vi "util.file.vars.vi"(4 "Operation(Read)":enum16{"Read File", "Write File"}(ring), 6 "allowDialogs?(False)":bool, 8 "error in":errorcluster, 9 "Directory (DIR_PROC)":T1, 10 "Proc Name(open dialog if empty)":string, 11 "Vars[] in":variant[](array[variant])) -> (0 "error out":errorcluster, 1 "filename":string, 2 "cancelled?":bool, 3 "Vars[] out":variant[](array[variant]), 5 "File path":path)   [LabVIEW 2024]
uses:
  controls/typePathSelector.ctl
  controls/typeProcVarientName.ctl
  Polymorphics/variantCtrlString.vi
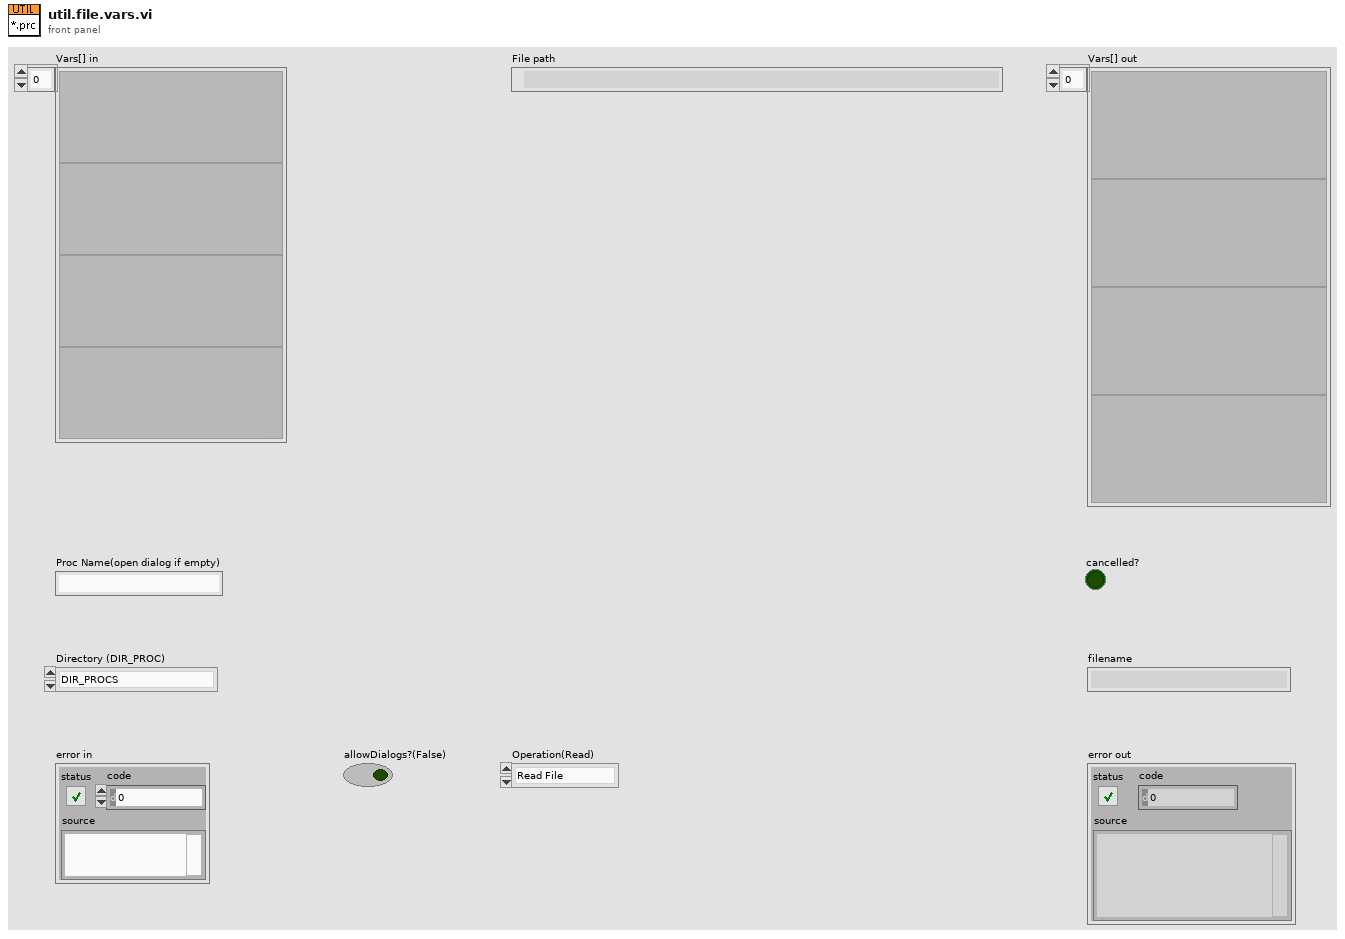
[diagram p1: front panel]
types:
  T1 = typedef "typePathSelector.ctl" = enum16{"DIR_PROCS", "DIR_CONFIG", "DIR_TEMPLATE", "DIR_IO_FILE", "DIR_RECORD", "DIR_LOG", "DIR_RUNTIME", "DIR_PRESET", "DIR_INI"}
  T2 = typedef "typeProcVarientName.ctl" = enum16{"procNameID", "procModuleID", "procPath", "procIsRunning", "procIndex", "procModule", "procRegisterNumeric", "procRegisterString", "procReport", "procReportPrev", "procCLK", "procStepPointer", "procType"}
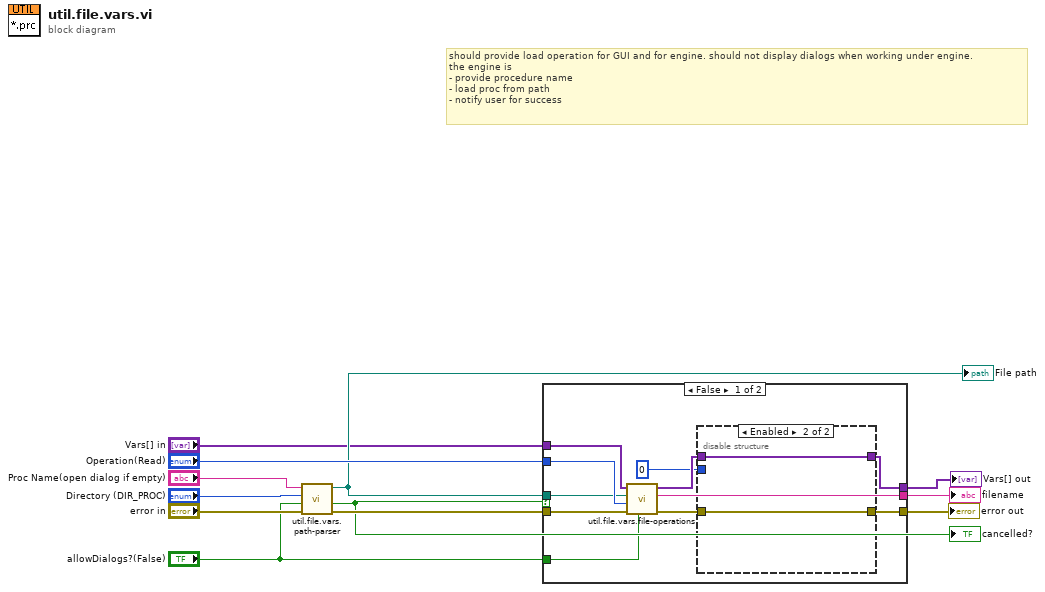
[diagram p0: block diagram]
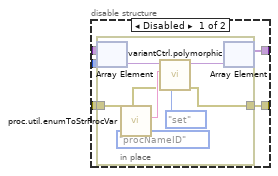
[diagram p2: hidden frame]
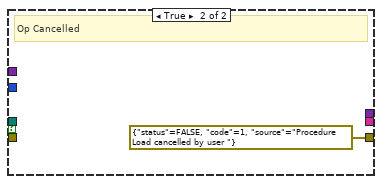
[diagram p3: hidden frame]
diagram:
  # "should provide load operation for GUI and for engine. should not display dialogs when working under engine.\nthe engine is\n- provide procedure name  \n- load proc from path\n- notify user for success"
  n1 = call "util.file.vars.path-parser.vi"("error in (no error)"="error in", "allowDialogs?(False)"="allowDialogs?(False)", "location (PROCEDURE_DIR)"="Directory (DIR_PROC)", "Proc name"="Proc Name(open dialog if empty)") -> ("error out"=w12:errorcluster, "cancelled"=w4:bool, "selected path"=w5:path)  [unwired: 5 in]
  "cancelled?" <- w4
  "File path" <- w5
  n2 = case shown="False" w4 {
    tunnel: [w23 _] -> w2
    tunnel: w12 -> [w22 _]
    tunnel: w5 -> [w18 _]
    tunnel: [w13 errorcluster {"status"=FALSE, "code"=1, "source"="Procedure Load cancelled by user "} ("error out")] -> w10
    tunnel: "Operation(Read)" -> [w21 _]
    tunnel: "allowDialogs?(False)" -> [w20 _]
    tunnel: [w16 _] -> w1
    tunnel: "Vars[] in" -> [w19 _]
    frame False {
      n3 = call "util.file.vars.file-operations.vi"("allowDialogs?(False)"=w20, "error in (no error)"=w22, "Operation(Read)"=w21, "selected path"=w18, "Vars[] in"=w19) -> ("error out"=w14:errorcluster, "filename"=w23:string, "Procedure"=w17:variant[])  [unwired: 4 in]
      n4 = disable-structure shown="Enabled" {
        disable-tunnel: w17 -> [w28 w37]
        disable-tunnel: [w27 w37] -> w16
        disable-tunnel: 0 -> [w26 _]
        disable-tunnel: w14 -> [w25 w36]
        disable-tunnel: [w24 w36] -> w13
        frame Disabled {
          n5 = in-place {
            in-place-border: w25 -> [w31]
            in-place-border: [w30] -> w24
            n6 = in-place-array #1(w28, w26) -> (w33:variant)
            n7 = call "proc.util.enumToStrProcVar.vi"("Proc var"=typeProcVarientName."procNameID") -> ("String"=w35:string)  [unwired: 10 in]
            n8 = call-poly "variantCtrl.polymorphic.vi"("menu in (get)"=enum16{"get", "set"}."set", "error in"=w31, "name in"=w35, "Step in"=w33) -> ("error out"=w30:errorcluster, "Step out"=w32:variant)  [unwired: 4 in, 2 out]
            n9 = in-place-array #1(w32) -> (w27:variant[])  [unwired: 1 out]
          }
        }
        frame Enabled {
        }
      }
    }
    frame True {
      # "Op Cancelled"
    }
  }
  "Vars[] out" <- w1
  "error out" <- w10
  "filename" <- w2
